vi "case.vi"() -> ()   [LabVIEW 2017]
panel:
  in  "String":string
  in  "Ring":u16(ring) items=["C", "F", "R"]
  out "Температура":dbl
  # "C F R"
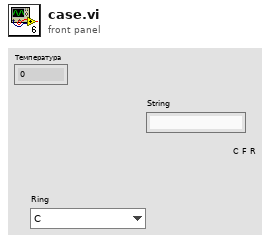
[diagram p1: front panel]
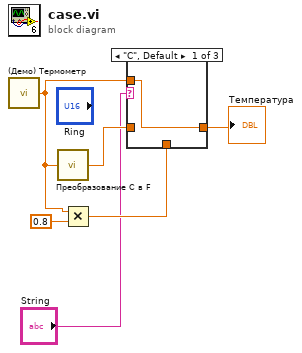
[diagram p0: block diagram]
diagram:
  n1 = call "(Демо) Термометр.vi"() -> ("Температура"=w3:dbl)  [unwired: 1 in]
  n2 = call "Преобразование C в F.vi"("Град C"=w3) -> ("Град F"=w6:dbl)
  n3 = Multiply(x=w3, y=0.8) -> (x*y=w2:dbl)
  n4 = case shown="\"C\", Default" "String" {
    tunnel: w6 -> [_ w8 _]
    tunnel: [w7 w8 w9] -> w5
    tunnel: w3 -> [w7 _ _]
    tunnel: w2 -> [_ _ w9]
    frame "C", Default {
    }
    frame "F" {
    }
    frame "R" {
    }
  }
  "Температура" <- w5
